vi "Report.vi"(6 "文件重命名":bool, 7 "文件名称":string, 8 "错误输入（无错误）":errorcluster, 11 "检测结果":bool[][](array[boolean])=[[TRUE]]) -> (0 "error out":errorcluster caption="错误输出", 3 "PRODUCT_VAULE":string)   [LabVIEW 2020]
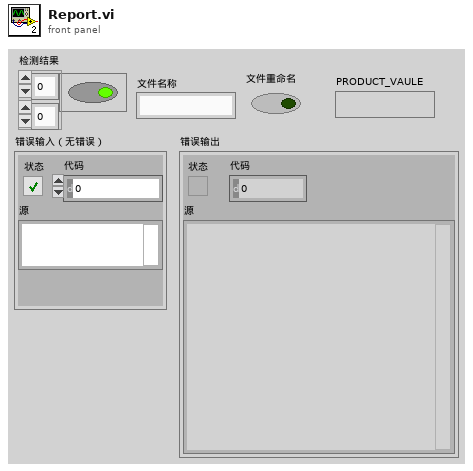
[diagram p1: front panel]
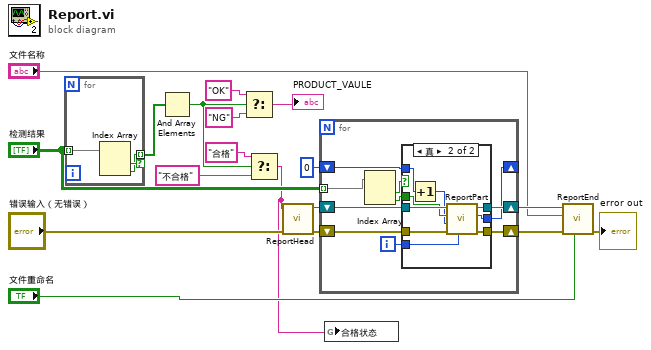
[diagram p0: block diagram]
diagram:
  n1 = for {
    tunnel: [w19] -> w4 mode=indexing if=w20
    tunnel: "检测结果" -> [w21] mode=indexing
    n2 = Index Array(array=w21) -> (element #1=w20:bool, element #2=w19:bool)  [unwired: 2 in]
  }
  n3 = And Array Elements(Boolean array=w4) -> (logical AND=w5:bool)
  n4 = Select(t="OK", s=w5, f="NG") -> (s? t:f=→"PRODUCT_VAULE":string)
  n5 = Select(t="合格", s=w5, f="不合格") -> (s? t:f=w1:string)
  n6 = call "ReportHead.vi"("error in (no error)"="错误输入（无错误）", "产品状态"=w1) -> ("error out"=w17:errorcluster, "report out"=w18:refnum<class "NI_report.lvclass">)  [unwired: 8 in]
  n7 = for {
    shift-right: [w29] -> w16
    shift-left: w18 -> [w31]
    shift-right: [w28] -> w15
    shift-left: w17 -> [w30]
    tunnel: "检测结果" -> [w24] mode=indexing
    shift-right: [w25] -> _
    shift-left: 0 ("索引OUT") -> [w26]
    i -> [w27]
    n8 = Index Array(array=w24) -> (element #1=w23:bool, element #2=w22:bool)  [unwired: 2 in]
    n9 = case shown="真" w23 {
      tunnel: w31 -> [w33 w43]
      tunnel: w30 -> [w34 w42]
      tunnel: [w33 w41] -> w29
      tunnel: [w34 w40] -> w28
      tunnel: w27 -> [_ w39]
      tunnel: w22 -> [_ w38]
      tunnel: w26 -> [w32 w36]
      tunnel: [w32 w37] -> w25
      frame False {
      }
      frame True {
        n10 = Increment(x=w36) -> (x+1=w35:i32)
        n11 = call "ReportPart.vi"("试验项目"=w39, "error in"=w42, "索引IN"=w35, "合格"=w38, "report in"=w43) -> ("error out 2"=w40:errorcluster, "索引OUT"=w37:i32, "report out"=w41:refnum<class "NI_report.lvclass">)  [unwired: 4 in]
      }
    }
  }
  n12 = global write "检测结果.vi" "合格状态"(w1) -> ()
  n13 = call "ReportEnd.vi"("文件重命名"="文件重命名", "error in (no error)"=w15, "文件名称"="文件名称", "report in"=w16) -> ("error out"=→"error out":errorcluster)  [unwired: 7 in]
